vi "SetDefaults.vi"(8 "error in (no error)":errorcluster, 11 "ArgparseWrapper in":refnum<class "ArgparseWrapper.lvclass">) -> (0 "error out":errorcluster, 3 "ArgparseWrapper out":refnum<class "ArgparseWrapper.lvclass">)   [LabVIEW 2022 SP3, in "ArgumentParser.lvlib" / "ArgparseWrapper.lvclass"]
uses:
  ArgparseWrapper.lvclass
  PythonWrapper/Source/PythonWrapper/PythonWrapper.lvclass
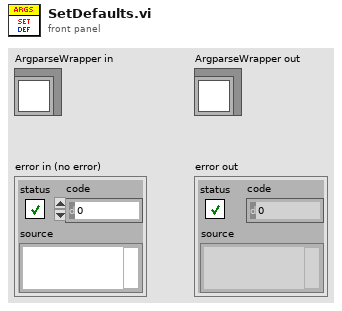
[diagram p1: front panel]
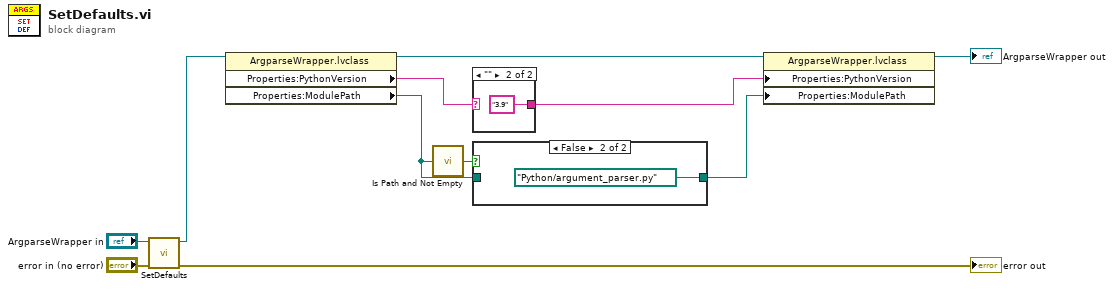
[diagram p0: block diagram]
diagram:
  n1 = call-parent "SetDefaults.vi"("error in (no error)"="error in (no error)", "PythonWrapper in"="ArgparseWrapper in") -> ("error out"=→"error out":errorcluster, "PythonWrapper out"=w2:refnum<class "ArgparseWrapper.lvclass">)  [unwired: 8 in]
  n2 = property class="ArgparseWrapper.lvclass"(reference=w2) -> (reference out=w8:refnum<class "ArgparseWrapper.lvclass">, "Properties:PythonVersion"=w3:string, "Properties:ModulePath"=w6:path)  [unwired: 1 in, 1 out]
  n3 = call <vilib>:"Is Path and Not Empty.vi"("path"=w6) -> ("Is Path and Not Empty?"=w7:bool)  [unwired: 4 in]
  n4 = case shown="\"\"" w3 {
    selector: w3 -> [w12 _]
    tunnel: [w12 "3.9" ("PythonVersion")] -> w4
    frame Default {
    }
    frame "" {
    }
  }
  n5 = case shown="False" w7 {
    tunnel: [w14 path "Python/argument_parser.py" ("ModulePath")] -> w5
    tunnel: w6 -> [w14 _]
    frame True {
    }
    frame False {
    }
  }
  n6 = property class="ArgparseWrapper.lvclass"(reference=w8, "Properties:PythonVersion"=w4, "Properties:ModulePath"=w5) -> (reference out=→"ArgparseWrapper out":refnum<class "ArgparseWrapper.lvclass">)  [unwired: 1 in, 1 out]
